vi "SerialCall.vi"(8 "error in (no error)":errorcluster, 10 "data":T1[](array[typedef]), 11 "Resource":string) -> (0 "error out":errorcluster, 3 "Response":string)   [LabVIEW 2013, in "Advanced Plotting Toolkit.lvlib"]
uses:
  Advanced Plotting Toolkit.lvlib
  KeyValue.ctl
  kernel32.dll
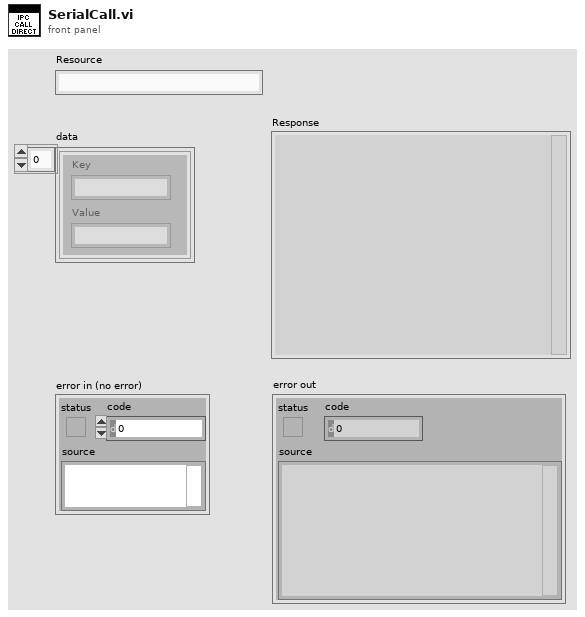
[diagram p1: front panel]
types:
  T1 = typedef "Advanced Plotting Toolkit.lvlib/KeyValue.ctl" = cluster{"Key":string, "Value":string}
  T2 = enum16{"big-endian, network order", "native, host order", "little-endian"}
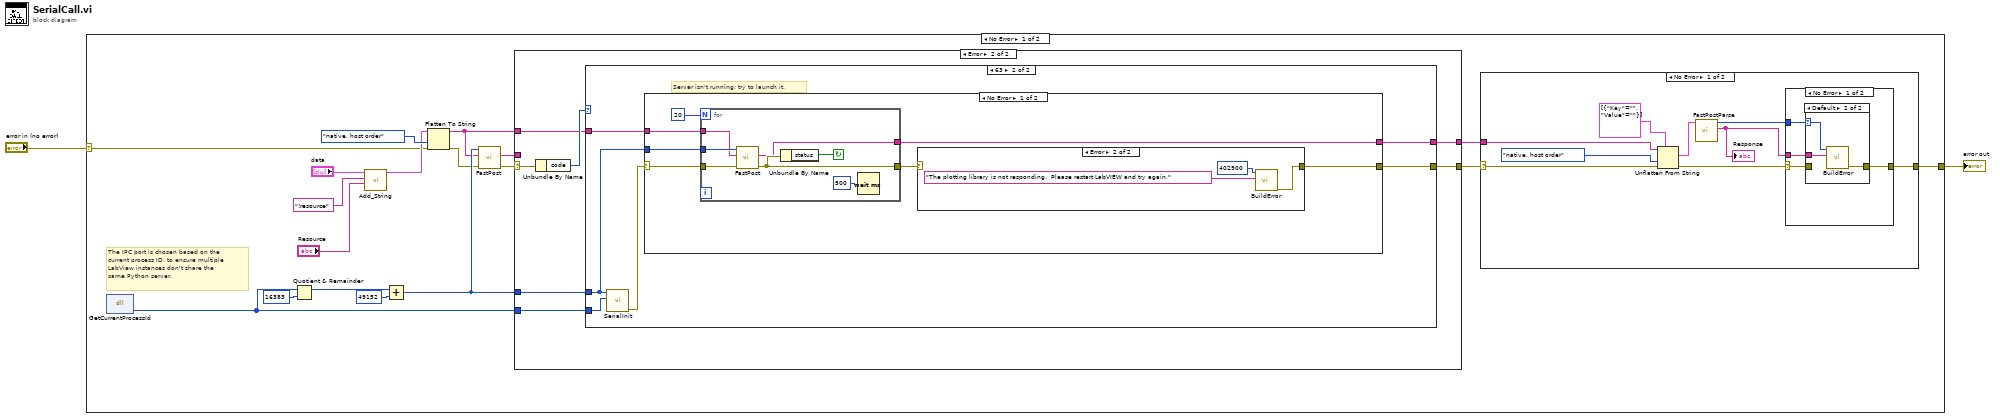
[diagram p0: block diagram]
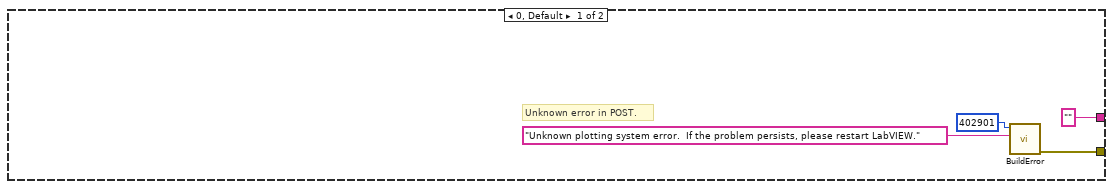
[diagram p6: hidden frame]
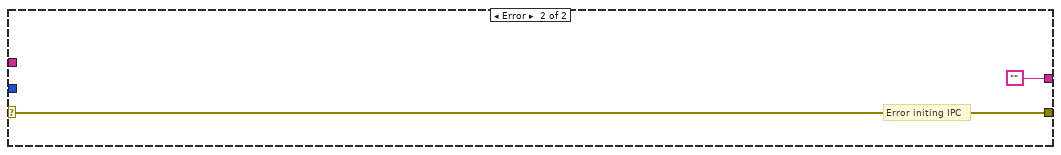
[diagram p8: hidden frame]
diagram:
  n1 = case shown="No Error" "error in (no error)" {
    selector: "error in (no error)" -> [w4 w79]
    tunnel: [w6 w79] -> w2
    frame No Error {
      # "The IPC port is chosen based on the\ncurrent process ID, to ensure multiple\nLabView instances don't share the\nsame Python server."
      n2 = dll-call lib="kernel32.dll" fn="GetCurrentProcessId"() -> ("return type"=w3:u32)  [unwired: 3 in, 2 out]
      n3 = Quotient & Remainder(x=w3, y=u32 16383) -> (x-y*floor(x/y)=w19:u32)  [unwired: 1 out]
      n4 = call "Add_String.vi"("Value"="Resource", "Key"="!resource", "Keyword Array"="data") -> ("Keyword Array Out"=w7:T1[])  [unwired: 8 in]
      n5 = Add(x=w19, y=49152) -> (x+y=w14:u32)
      n6 = Flatten To String(anything=w7, byte order (0:big-endian, network order)=T2."native, host order", error in (no error)=w4) -> (data string=w13:string, error out=w5:errorcluster)  [unwired: 1 in, 1 out]
      n7 = call "FastPost.vi"("error in (no error)"=w5, "Outbound"=w13, "IPC"=w14) -> ("error out"=w16:errorcluster, "Inbound"=w15:string)  [unwired: 7 in]
      n8 = case shown="Error" w16 {
        selector: w16 -> [w40 w48]
        tunnel: w15 -> [w41 _]
        tunnel: w14 -> [_ w46]
        tunnel: w13 -> [_ w45]
        tunnel: [w41 w44] -> w11
        tunnel: [w40 w43] -> w12
        tunnel: w3 -> [_ w42]
        frame No Error {
        }
        frame Error {
          n9 = Unbundle By Name(w48) -> ("code"=w47:i32)
          n10 = case shown="63" w47 {
            tunnel: w46 -> [_ w57]
            tunnel: w45 -> [_ w56]
            tunnel: ["" ("Inbound") w55] -> w44
            tunnel: [w50 w54] -> w43
            tunnel: w42 -> [_ w53]
            frame 0, Default {
              # "Unknown error in POST."
              n11 = call "BuildError.vi"("Source"="Unknown plotting system error.  If the problem persists, please restart LabVIEW." ("error message (\"\")"), "Code"=402901 ("error code (0)")) -> ("error out"=w50:errorcluster)  [unwired: 9 in]
            }
            frame 63 {
              # "Server isn't running; try to launch it."
              n12 = call "SerialInit.vi"("PID"=w53, "IPC"=w57) -> ("error out"=w58:errorcluster)  [unwired: 9 in]
              n13 = case shown="No Error" w58 {
                selector: w58 -> [w64 w78]
                tunnel: [w59 w78] -> w54
                tunnel: w57 -> [w63 _]
                tunnel: w56 -> [w62 _]
                tunnel: [w61 ""] -> w55
                frame No Error {
                  n14 = for {
                    N: 20 -> [_]
                    tunnel: w63 -> [w72]
                    tunnel: w62 -> [w71]
                    tunnel: [w70] -> w61
                    tunnel: w64 -> [w74]
                    tunnel: [w73] -> w60
                    stop <- w75 continue-if-true
                    n15 = call "FastPost.vi"("error in (no error)"=w74, "Outbound"=w71, "IPC"=w72) -> ("error out"=w73:errorcluster, "Inbound"=w70:string)  [unwired: 7 in]
                    n16 = Unbundle By Name(w73) -> ("status"=w75:bool)
                    n17 = Wait (ms)(milliseconds to wait=u32 500) -> ()  [unwired: 1 out]
                  }
                  n18 = case shown="Error" w60 {
                    selector: w60 -> [w66 _]
                    tunnel: [w66 w69] -> w59
                    frame No Error {
                    }
                    frame Error {
                      n19 = call "BuildError.vi"("Source"="The plotting library is not responding.  Please restart LabVIEW and try again.", "Code"=402900) -> ("error out"=w69:errorcluster)  [unwired: 9 in]
                    }
                  }
                }
                frame Error {
                  # "Error initing IPC"
                }
              }
            }
          }
        }
      }
      n20 = case shown="No Error" w12 {
        selector: w12 -> [w25 w39]
        tunnel: w11 -> [w29 _]
        tunnel: [w21 w39] -> w6
        frame No Error {
          n21 = Unflatten From String(type=T1[] [{"Key"="", "Value"=""}], binary string=w29, byte order (0:big-endian, network order)=T2."native, host order", error in (no error)=w25) -> (value=w26:T1[], error out=w24:errorcluster)  [unwired: 1 in, 1 out]
          n22 = call "FastPostParse.vi"("Data"=w26) -> ("Body"=w22:string, "Status"=w23:i32)  [unwired: 9 in]
          "Response" <- w22
          n23 = case shown="No Error" w24 {
            selector: w24 -> [w32 w38]
            tunnel: w23 -> [w33 _]
            tunnel: w22 -> [w31 _]
            tunnel: [w30 w38] -> w21
            frame No Error {
              n24 = case shown="Default" w33 {
                selector: w33 -> [_ w37]
                tunnel: w32 -> [w34 _]
                tunnel: [w34 w35] -> w30
                tunnel: w31 -> [_ w36]
                frame 0 {
                }
                frame Default {
                  n25 = call "BuildError.vi"("Source"=w36, "Code"=w37) -> ("error out"=w35:errorcluster)  [unwired: 9 in]
                }
              }
            }
            frame Error {
            }
          }
        }
        frame Error {
        }
      }
    }
    frame Error {
    }
  }
  "error out" <- w2
